vi "disable_DAC.vi"() -> ()   [LabVIEW 2014]
uses:
  aardvark.dll
panel:
  out "DAC Current State":bool[](array[boolean])
  in  "DAC":bool[](array[boolean])
  in  "Address (0x50)":u16=80 max=1023 format="%.0x"
  in  "Num Bytes to Fetch (64)":u16=64 min=1
  in  "Aardvark Handle":i32 min=0
  out "error out":errorcluster
  in  "error in (no error)":errorcluster
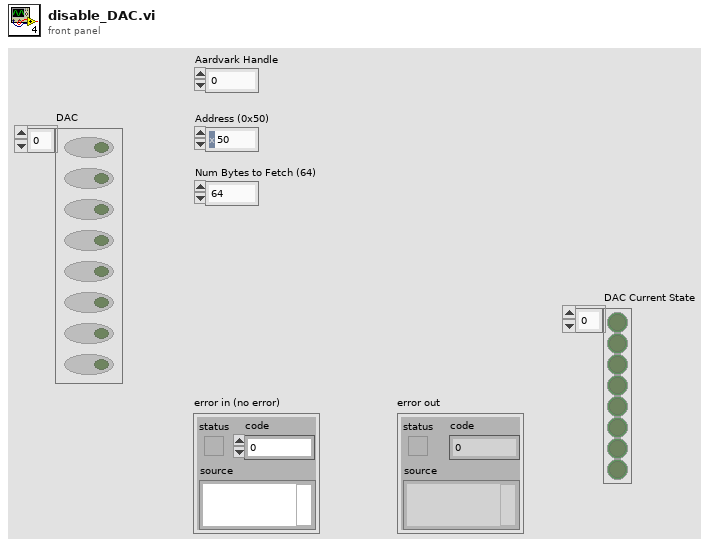
[diagram p1: front panel]
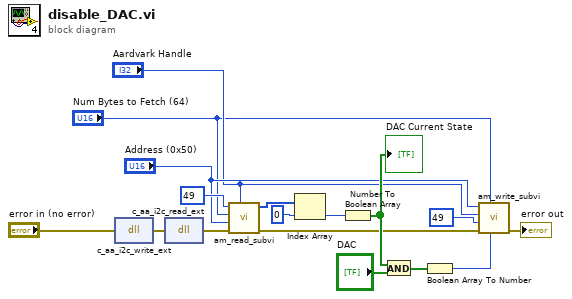
[diagram p0: block diagram]
diagram:
  n1 = dll-call lib="C:/Users/p282652/Documents/LabVIEW Data/Demonstrator/labviewFunctions_AM/aardvark.dll" fn="c_aa_i2c_write_ext"(error in="error in (no error)") -> (error out=w11:errorcluster)  [unwired: 3 in, 1 out]
  n2 = dll-call lib="C:/Users/p282652/Documents/LabVIEW Data/Demonstrator/labviewFunctions_AM/aardvark.dll" fn="c_aa_i2c_read_ext"(error in=w11) -> (error out=w9:errorcluster)  [unwired: 3 in, 1 out]
  n3 = call "am_read_subvi.vi"("Aardvark Handle in"="Aardvark Handle", "error in (no error)"=w9, "Address (0x50) in"="Address (0x50)", "Num Bytes to Fetch (64)"="Num Bytes to Fetch (64)", "Memory ADD"=u16 49) -> ("error out"=w4:errorcluster, "Array"=w8:u8[])  [unwired: 5 in]
  n4 = Index Array(array=w8, index=0) -> (element=w16:u8)
  n5 = Number To Boolean Array(number=w16) -> (Boolean array=w14:bool[])
  "DAC Current State" <- w14
  n6 = And(x=w14, y="DAC") -> (x .and. y?=w13:bool[])
  n7 = Boolean Array To Number(Boolean array=w13) -> (number=w2:u32)
  n8 = call "am_write_subvi.vi"("Data to Write"=w2, "Num Bytes to Fetch (64)"="Num Bytes to Fetch (64)", "error in (no error)"=w4, "Memory ADD"=u16 49, "Aardvark Handle in"="Aardvark Handle", "Address (0x50) in"="Address (0x50)") -> ("error out"=→"error out":errorcluster)  [unwired: 4 in, 1 out]
